vi "tcsOfc_getSample_degreeOfFreedom.vi"(8 "error in (no error)":errorcluster, 11 "degreeOfFreedom_Ctl":T1={"dof[50]"=[0.0, 0.0, 0.0, 0.0, 0.0, 0.0, 0.0, 0.0, 0.0, 0.0, 0.0, 0.0, 0.0, 0.0, 0.0, 0.0, 0.0, 0.0, 0.0, 0.0, 0.0, 0.0, 0.0, 0.0, 0.0, 0.0, 0.0, 0.0, 0.0, 0.0, 0.0, 0.0, 0.0, 0.0, 0.0, 0.0, 0.0, 0.0, 0.0, 0.0, 0.0, 0.0, 0.0, 0.0, 0.0, 0.0, 0.0, 0.0, 0.0, 0.0]}) -> (0 "error out":errorcluster, 2 "function return":i32, 3 "degreeOfFreedom_Ctl out":T1)   [LabVIEW 2016, in "SALLV_tcsOfc.lvlib"]
doc: "int tcsOfc_shm_getSample_degreeOfFreedomLV(tcsOfc_degreeOfFreedomLV *degreeOfFreedom_Ctl );"
uses:
  SALLV_tcsOfc.lvlib
  DataTypes/degreeOfFreedom.ctl
  SALLV_tcsOfc.so
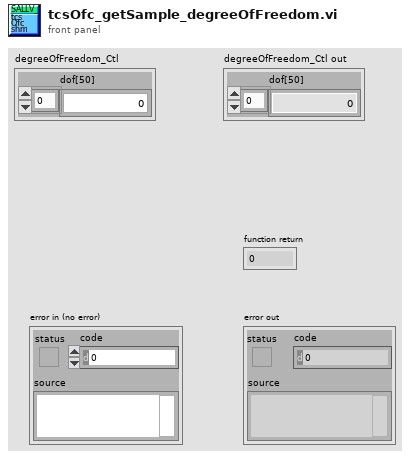
[diagram p1: front panel]
types:
  T1 = typedef "SALLV_tcsOfc.lvlib/degreeOfFreedom.ctl" = cluster{"dof[50]":dbl[]}
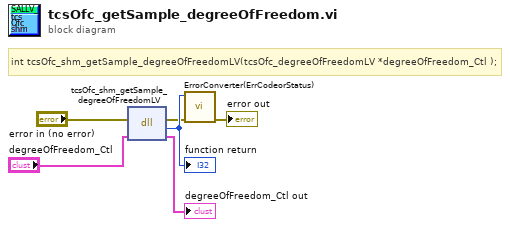
[diagram p0: block diagram]
diagram:
  # "int tcsOfc_shm_getSample_degreeOfFreedomLV(tcsOfc_degreeOfFreedomLV *degreeOfFreedom_Ctl );"
  n1 = dll-call lib="home/andres/Desktop/SAL_tcsOfc/SALLV_tcsOfc.*" fn="tcsOfc_shm_getSample_degreeOfFreedomLV"(error in="error in (no error)", "degreeOfFreedom_Ctl"="degreeOfFreedom_Ctl") -> (error out=w2:errorcluster, w6:i32, "degreeOfFreedom_Ctl"=→"degreeOfFreedom_Ctl out":T1)  [unwired: 2 in, 1 out]
  "function return" <- w6
  n2 = call "ErrorConverter(ErrCodeorStatus).vi"("error in (no error)"=w2, "error code"=w6) -> ("error out"=→"error out":errorcluster)  [unwired: 9 in]
